vi "PowerUp.vi"(0 "SMU Handle":refnum<k15>="PXI1Slot2", 1 "Current Limit  DxBoot0":dbl, 2 "Voltage Level DxBoot0":dbl, 7 "DxBoot0":string="0", 9 "DxSupply":string="0", 11 "error in (no error)":errorcluster, 12 "Current Limit DxSupply":dbl, 13 "Voltage Level DxSupply":dbl) -> (4 "IVI Refnum out":refnum<k15>, 15 "error out":errorcluster)   [LabVIEW 2018]
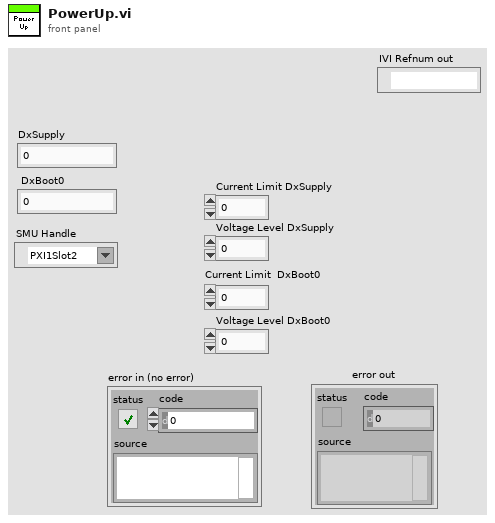
[diagram p1: front panel]
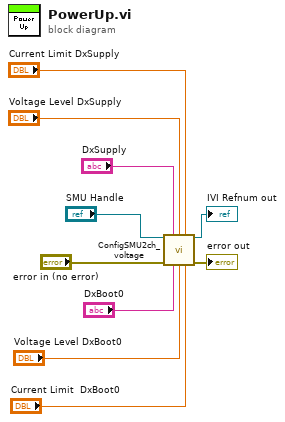
[diagram p0: block diagram]
diagram:
  n1 = call "ConfigSMU2ch_voltage.vi"("IVI Refnum in"="SMU Handle", "Channel DxSupply"="DxSupply", "Voltage Level DxSupply"="Voltage Level DxSupply", "Current Limit DxSupply"="Current Limit DxSupply", "error in (no error)"="error in (no error)", "Channel DxBoot0"="DxBoot0", "Voltage Level DxBoot0"="Voltage Level DxBoot0", "Current Limit DxBoot0"="Current Limit  DxBoot0") -> ("IVI Refnum out"=→"IVI Refnum out":refnum<k15>, "error out"=→"error out":errorcluster)  [unwired: 6 in]
